vi "Deselect Apps.vi"(8 "error in (no error)":errorcluster, 11 "AppListPanel in":refnum<class "AppListPanel.lvclass">) -> (0 "error out":errorcluster, 3 "AppListPanel out":refnum<class "AppListPanel.lvclass">)   [LabVIEW 2020, in "PicoG-App.lvlib" / "AppListPanel.lvclass"]
uses:
  AppListPanel.lvclass
  AppListPanel.lvclass/AppListPanel.ctl
  GWebAppArrayPanel/GWebAppArrayPanel.lvclass
  <vilib>/IlluminatedG/IG OOPanel/OOPanel/ArrayManager/ArrayManager.lvclass
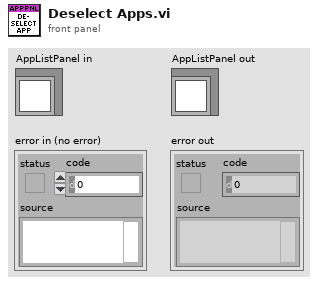
[diagram p1: front panel]
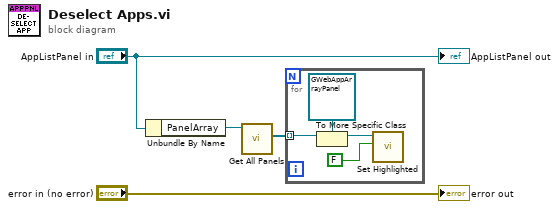
[diagram p0: block diagram]
diagram:
  n1 = Unbundle By Name("AppListPanel in") -> ("PanelArray"=w2:refnum<class "ArrayManager.lvclass">)
  n2 = call <vilib>:"Get All Panels.vi"("PanelArray in"=w2) -> ("Panels"=w1:refnum<class "ArrayPanel.lvclass">[])  [unwired: 8 in, 2 out]
  n3 = for {
    tunnel: w1 -> [w8] mode=indexing
    n4 = To More Specific Class(target class=refnum<class "GWebAppArrayPanel.lvclass"> refnum ("PicoG-App.lvlib:GWebAppArrayPanel.lvclass"), reference=w8) -> (specific class reference=w6:refnum<class "GWebAppArrayPanel.lvclass">)  [unwired: 1 in, 1 out]
    n5 = call "Set Highlighted.vi"("Highlighted"=FALSE, "GWebAppArrayPanel in"=w6) -> ()  [unwired: 8 in, 2 out]
  }
  "error out" <- "error in (no error)"
  "AppListPanel out" <- "AppListPanel in"
